vi "SVPO Scale Voltage to EU.vi"   [LabVIEW 2017, in "SoundVib_Calibration.lvlib"]
doc: "Scales the single-precision <B>signal [V]</B> from volts to the engineering units (EU) you select. Scale signals to appropriate EU before applying limits, saving to disk, and performing measurement analyses. Use this VI on embedded targets that have limited computational resources. Wire data to the <B>signal [V]</B> input to determine the polymorphic instance to use or manually select the instance."
uses:
  <vilib>/addons/Sound and Vibration/svt_Calibration/SoundVib_Calibration.lvlib
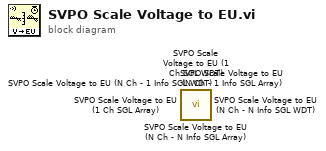
[diagram p0: block diagram]
diagram:
  n1 = call <vilib>:"SVPO Scale Voltage to EU (N Ch - N Info SGL Array).vi"() -> ()  [unwired: 10 in, 2 out]
  n2 = call <vilib>:"SVPO Scale Voltage to EU (N Ch - 1 Info SGL Array).vi"() -> ()  [unwired: 10 in, 2 out]
  n3 = call <vilib>:"SVPO Scale Voltage to EU (1 Ch SGL Array).vi"() -> ()  [unwired: 10 in, 2 out]
  n4 = call <vilib>:"SVPO Scale Voltage to EU (N Ch - N Info SGL WDT).vi"() -> ()  [unwired: 11 in, 1 out]
  n5 = call <vilib>:"SVPO Scale Voltage to EU (N Ch - 1 Info SGL WDT).vi"() -> ()  [unwired: 11 in, 1 out]
  n6 = call <vilib>:"SVPO Scale Voltage to EU (1 Ch SGL WDT).vi"() -> ()  [unwired: 11 in, 1 out]
